vi "ObtainQueue.vi"(6 "ModuleNumber":i32, 8 "error in (no error)":errorcluster, 10 "ModuleName":string) -> (0 "error out":errorcluster, 3 "MessageQueue":refnum<queue>)   [LabVIEW 2014, in "SyncModule.lvlib"]
uses:
  SyncModule.lvlib
  PublicAPI/Arguments/Messages/clMessage.ctl
panel:
  # "This obtains a queue and\nenqueues the \"Initialize\"\nMessage"
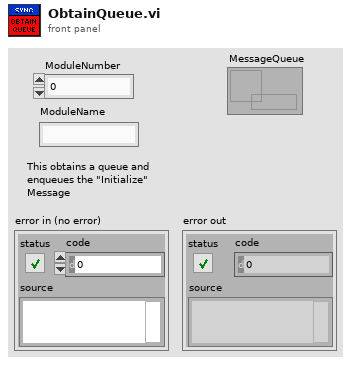
[diagram p1: front panel]
types:
  T1 = typedef "SyncModule.lvlib/clMessage.ctl" = cluster{"Message":string, "Message Data":variant}
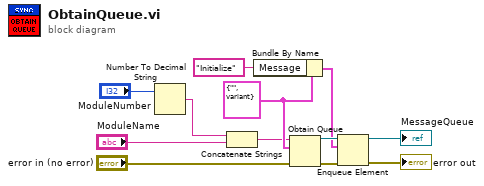
[diagram p0: block diagram]
diagram:
  w10 = T1 {"Message"="", "Message Data"=variant} ("clMessage")
  n1 = Number To Decimal String(number="ModuleNumber") -> (decimal integer string=w1:string)  [unwired: 1 in]
  n2 = Concatenate Strings(w1, "ModuleName") -> (w4:string)
  n3 = Bundle By Name(cluster=w10, "Message"="Initialize") -> (w8:T1)
  n4 = Obtain Queue(name (unnamed)=w4, element data type=w10, error in (no error)="error in (no error)") -> (queue out=w11:refnum<queue>, error out=w7:errorcluster)  [unwired: 2 in, 1 out]
  n5 = Enqueue Element(queue=w11, element=w8, error in (no error)=w7) -> (queue out=→"MessageQueue":refnum<queue>, error out=→"error out":errorcluster)  [unwired: 1 in, 1 out]
